vi "Launcher.vi"   [LabVIEW 2018]
uses:
  <vilib>/Utility/sysdir.llb/System Directory Type.ctl
  Libraries/Application/Application.lvlib
types:
  T1 = typedef "System Directory Type.ctl" = i32
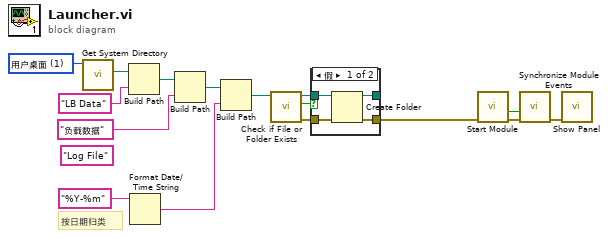
[diagram p0: block diagram]
diagram:
  (unwired) "Log File" ("名称或相对路径")
  w13 = T1 1 items=["用户目录"=0, "用户桌面"=1, "用户文档"=2, "用户应用程序数据"=3, "用户设置"=4, "用户临时目录"=5, "公共文档"=6, "公共应用程序数据"=7, "公共设置"=8, "公共缓存"=13, "系统核心库"=9, "系统安装库"=10, "应用程序文件"=11, "启动盘根目录"=12] ("system directory type")
  # "按日期归类"
  n1 = call <vilib>:"Get System Directory.vi"("system directory type"=w13) -> ("system directory"=w12:path)  [unwired: 10 in]
  n2 = Build Path(base path=w12, name or relative path="LB Data" ("名称或相对路径")) -> (appended path=w5:path)
  n3 = Format Date/Time String(time format string (%c)="%Y-%m" ("时间格式字符串(%c)")) -> (date/time string=w9:string)  [unwired: 2 in]
  n4 = Build Path(base path=w5, name or relative path="负载数据" ("名称或相对路径")) -> (appended path=w3:path)
  n5 = Build Path(base path=w3, name or relative path=w9) -> (appended path=w2:path)
  n6 = call <vilib>:"Check if File or Folder Exists.vi"("path"=w2) -> ("error out"=w7:errorcluster, "file or folder exists?"=w8:bool, "dup path"=w6:path)  [unwired: 8 in]
  n7 = case shown="假" w8 {
    tunnel: w6 -> [w20 w21]
    tunnel: w7 -> [w19 w22]
    tunnel: [w18 w22] -> w1
    tunnel: [w17 w21] -> _
    frame False {
      n8 = Create Folder(path (use dialog)=w20, error in=w19) -> (created path=w17:path, error out=w18:errorcluster)  [unwired: 1 in, 1 out]
    }
    frame True {
    }
  }
  n9 = call "Start Module.vi"("error in"=w1) -> ("error out"=w15:errorcluster, "Wait for Event Sync?"=w16:bool)  [unwired: 7 in, 2 out]
  n10 = call "Synchronize Module Events.vi"("error in"=w15, "Wait for Event Sync?"=w16) -> ("error out"=w14:errorcluster)  [unwired: 9 in]
  n11 = call "Show Panel.vi"("error in (no error)"=w14) -> ()  [unwired: 10 in, 1 out]
